vi "Report init interface.vi"(8 "Fehler (Eingang, kein Fehler)":errorcluster, 10 "VI Referenz":refnum<vi>, 11 "SubPanel (Eingang)":refnum<vi>) -> (0 "Fehler (Ausgang)":errorcluster, 3 "Report out":refnum<class "Report.lvclass">)   [LabVIEW 2013]
uses:
  classes/Datastructure/Report/Report.lvclass
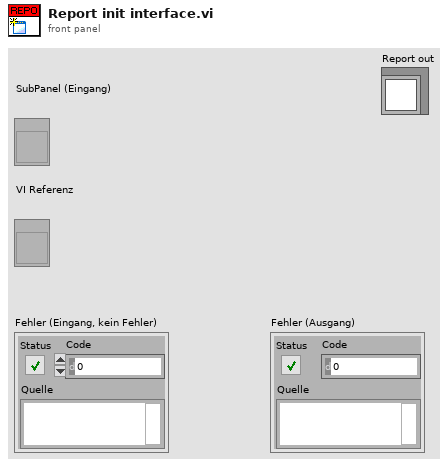
[diagram p1: front panel]
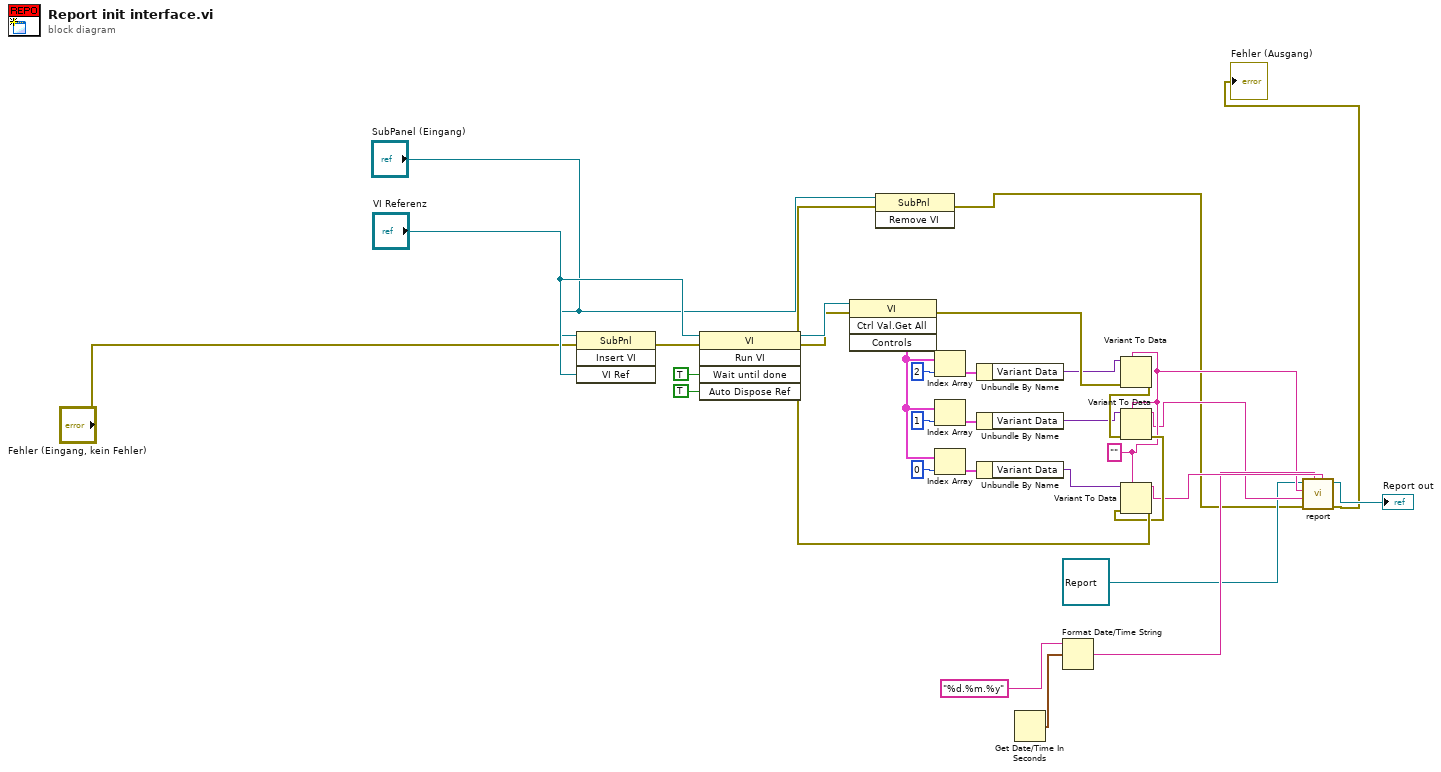
[diagram p0: block diagram]
diagram:
  w6 = ""
  n1 = invoke on="Invoke Node" class="SubPnl" method="Insert VI"(reference="SubPanel (Eingang)", error in="Fehler (Eingang, kein Fehler)", "VI Ref"="VI Referenz") -> (error out=w20:errorcluster)  [unwired: 1 in, 3 out]
  n2 = invoke on="Methodenknoten" class="VI" method="Run VI"(reference="VI Referenz", error in=w20, "Wait until done"=TRUE ("Warten bis beendet"), "Auto Dispose Ref"=TRUE ("Referenz automatisch schließen")) -> (reference out=w22:refnum<vi>, error out=w21:errorcluster)  [unwired: 1 in, 3 out]
  n3 = invoke class="VI" method="Ctrl Val.Get All"(reference=w22, error in=w21) -> (error out=w27:errorcluster, "Get All Control Values Variant"=w13:cluster{"Name":string, "Variant Data":variant}[])  [unwired: 2 in, 2 out]
  n4 = Index Array(array=w13, index=2) -> (element=w12:cluster{"Name":string, "Variant Data":variant})
  n5 = Index Array(array=w13, index=1) -> (element=w11:cluster{"Name":string, "Variant Data":variant})
  n6 = Index Array(array=w13, index=0) -> (element=w16:cluster{"Name":string, "Variant Data":variant})
  n7 = Unbundle By Name(w12) -> ("Variant Data"=w25:variant)
  n8 = Unbundle By Name(w11) -> ("Variant Data"=w26:variant)
  n9 = Unbundle By Name(w16) -> ("Variant Data"=w24:variant)
  n10 = Get Date/Time In Seconds() -> (seconds since 1Jan1904=w8:timestamp)
  n11 = Format Date/Time String(time format string (%c)="%d.%m.%y" ("Zeitformatierungs-String (%c)"), seconds (now)=w8) -> (date/time string=w7:string)  [unwired: 1 in]
  n12 = Variant To Data(error in=w27, type=w6, Variant=w25) -> (error out=w28:errorcluster)  [unwired: 1 out]
  n13 = Variant To Data(error in=w28, type=w6, Variant=w26) -> (data=w5:string, error out=w29:errorcluster)
  n14 = Variant To Data(error in=w29, type=w6, Variant=w24) -> (data=w10:string, error out=w30:errorcluster)
  n15 = invoke on="Invoke Node" class="SubPnl" method="Remove VI"(reference="SubPanel (Eingang)", error in=w30) -> (error out=w2:errorcluster)  [unwired: 1 in, 2 out]
  n16 = call-dynamic "report.vi"("Rname"=w10, "date"=w7, "error in (no error)"=w2, "pruefer"=w5, "obnr"=w6, "Report in"=refnum<class "Report.lvclass"> refnum) -> ("error out"=→"Fehler (Ausgang)":errorcluster, "Report out"=→"Report out":refnum<class "Report.lvclass">)  [unwired: 4 in]
